vi "N4_X01_write_range.vi"(0 "DriverConnect in":T1={"InterfaceType"=enum."VISA", "OpenedSession"="", "InterfaceSettings"={"Interface"=enum."RS232", "EOS 4 read"=enum."LF (\\n)", "EOS 4 write"=enum."LF (\\n)", "TMO, ms"=10000, "Sett"=variant(cluster{"Baud Rate":u32, "Data Bits":u16, "Parity":u16, "Stop Bits":u16, "Flow Control":u16, "Eho":bool} {"Baud Rate"=75, "Data Bits"=0, "Parity"=0, "Stop Bits"=0, "Flow Control"=0, "Eho"=FALSE})}}, 1 "Command range":T7, 2 "ModeIsChanged?":T6, 11 "error in":T8, 12 "Error Code":T10, 14 "Driver Name":T9) -> (4 "DriverConnect out":T1={"InterfaceType"=enum."VISA", "OpenedSession"="", "InterfaceSettings"={"Interface"=enum."RS232", "EOS 4 read"=enum."LF (\\n)", "EOS 4 write"=enum."LF (\\n)", "TMO, ms"=10000, "Sett"=variant(cluster{"Baud Rate":u32, "Data Bits":u16, "Parity":u16, "Stop Bits":u16, "Flow Control":u16, "Eho":bool} {"Baud Rate"=75, "Data Bits"=0, "Parity"=0, "Stop Bits"=0, "Flow Control"=0, "Eho"=FALSE})}}, 8 "RangeWasChanged":T6=TRUE, 15 "error out":T8)   [LabVIEW 2018]
uses:
  MOKO_LabViewLibrary/MokoLowLevel/MokoLowLovelControl/MLLC_ErrorCode.ctl
  MOKO_LabViewLibrary/MokoLowLevel/MokoLowLovelControl/MLLC_DriverName.ctl
  MOKO_LabViewLibrary/MokoLowLevel/MokoLowLovelControl/MLLC_Error.ctl
  MOKO_LabViewLibrary/MokoLowLevel/MokoLowLovelControl/MLLC_Command.ctl
  MOKO_LabViewLibrary/MokoLowLevel/MokoLowLovelControl/MLLC_Boolean.ctl
  MOKO_LabViewLibrary/MokoLowLevel/MokoLowLovelControl/MLLC_ConnectCluster.ctl
  MOKO_LabViewLibrary/MokoLowLevel/MokoLowLovelControl/MLLC_InterfaceType.ctl
  MOKO_LabViewLibrary/MokoLowLevel/MokoLowLovelControl/MLLC_OpenedSession.ctl
  MOKO_LabViewLibrary/MokoLowLevel/MokoLowLovelControl/MLLC_InterfaceSettings.ctl
  MOKO_LabViewLibrary/MokoLowLevel/MokoLowLovelControl/MLLC_InterfaceKind.ctl
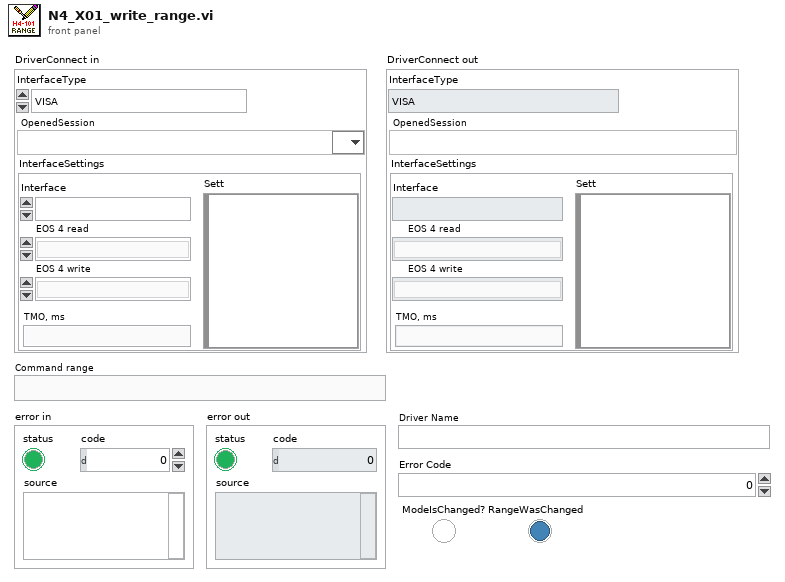
[diagram p1: front panel]
types:
  T1 = typedef "MLLC_ConnectCluster.ctl" = cluster{"InterfaceType":T2, "OpenedSession":T3, "InterfaceSettings":T4}
  T2 = typedef "MLLC_InterfaceType.ctl" = enum16{"VISA", "Prologix USB-GPIB"}
  T3 = typedef "MLLC_OpenedSession.ctl" = refnum<visa-resource-name>
  T4 = typedef "MLLC_InterfaceSettings.ctl" = cluster{"Interface":T5, "EOS 4 read":enum16{"Default (=EOS 4 write)", "CR (\\r)", "LF (\\n)", "None"}, "EOS 4 write":enum16{"CR+LF (\\r\\n)", "CR (\\r)", "LF (\\n)", "None"}, "TMO, ms":i32, "Sett":variant}
  T5 = typedef "MLLC_InterfaceKind.ctl" = enum16{"RS232", "GPIB", "USB", "Ethernet", "another"}
  T6 = typedef "MLLC_Boolean.ctl" = bool
  T7 = typedef "MLLC_Command.ctl" = string
  T8 = typedef "MLLC_Error.ctl" = errorcluster
  T9 = typedef "MLLC_DriverName.ctl" = string
  T10 = typedef "MLLC_ErrorCode.ctl" = u32
  T11 = typedef "MLLC_Response.ctl" = string
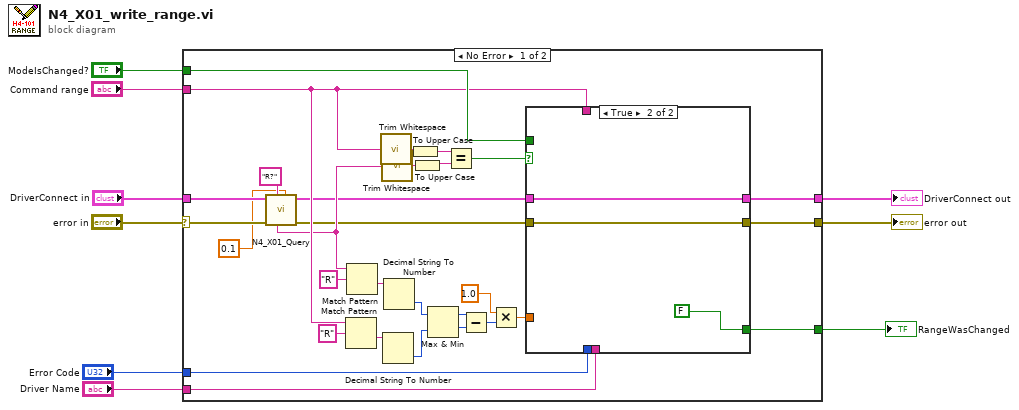
[diagram p0: block diagram]
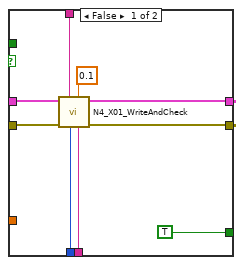
[diagram p2: hidden frame]
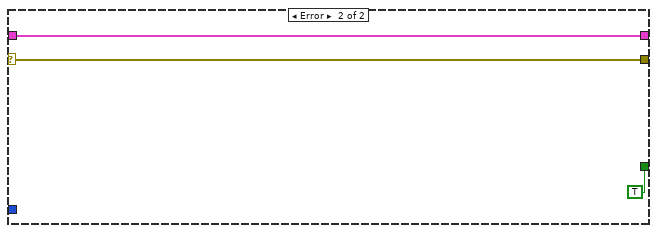
[diagram p3: hidden frame]
diagram:
  n1 = case shown="No Error" "error in" {
    selector: "error in" -> [w35 w54]
    tunnel: [w37 w54] -> w9
    tunnel: [w38 w53] -> w1
    tunnel: "Error Code" -> [w34 _]
    tunnel: "Driver Name" -> [w33 _]
    tunnel: "DriverConnect in" -> [w39 w53]
    tunnel: "Command range" -> [w31 _]
    tunnel: [w36 TRUE] -> w4
    tunnel: "ModeIsChanged?" -> [w32 _]
    frame No Error {
      n2 = call "N4_X01_Query.vi"("Delay Befor (s)"=0.1 ("Command Time (s)"), "Command"="R?" ("Error Query"), "error in"=w35, "DriverConnect in"=w39) -> ("error out"=w11:T8, "DriverConnect out"=w12:T1, "Response"=w13:T11)  [unwired: 5 in]
      n3 = Match Pattern(string=w31, regular expression="R") -> (after substring=w22:T7)  [unwired: 1 in, 3 out]
      n4 = Match Pattern(string=w13, regular expression="R") -> (after substring=w23:T11)  [unwired: 1 in, 3 out]
      n5 = call <vilib>:"Trim Whitespace.vi"("string"=w31) -> ("trimmed string"=w26:string)  [unwired: 1 in]
      n6 = call <vilib>:"Trim Whitespace.vi"("string"=w13) -> ("trimmed string"=w28:string)  [unwired: 1 in]
      n7 = Decimal String To Number(string=w22) -> (number=w19:i32)  [unwired: 2 in, 1 out]
      n8 = Decimal String To Number(string=w23) -> (number=w20:i32)  [unwired: 2 in, 1 out]
      n9 = To Upper Case(1:w26) -> (0:w27:string)
      n10 = To Upper Case(1:w28) -> (0:w29:string)
      n11 = Max & Min(x=w20, y=w19) -> (max(x,y)=w18:i32, min(x,y)=w17:i32)
      n12 = Equal?(x=w27, y=w29) -> (x = y?=w25:bool)
      n13 = Subtract(x=w18, y=w17) -> (x-y=w16:i32)
      n14 = Multiply(x=1.0 ("Delay Time (s)"), y=w16) -> (x*y=w15:dbl)
      n15 = case shown="True" w25 {
        tunnel: w34 -> [w48 _]
        tunnel: w33 -> [w47 _]
        tunnel: [w46 w51] -> w38
        tunnel: [w45 w50] -> w37
        tunnel: w31 -> [w44 _]
        tunnel: w12 -> [w41 w51]
        tunnel: w11 -> [w40 w50]
        tunnel: [TRUE FALSE] -> w36
        tunnel: w32 -> [_ _]
        tunnel: w15 -> [_ _]
        frame False {
          n16 = call "N4_X01_WriteAndCheck.vi"("Driver Name"=w47, "Command Time (s)"=0.1, "Error Code"=w48, "Command"=w44, "error in"=w40, "DriverConnect in"=w41) -> ("error out"=w45:T8, "DriverConnect out"=w46:T1)  [unwired: 4 in]
        }
        frame True {
        }
      }
    }
    frame Error {
    }
  }
  "error out" <- w9
  "RangeWasChanged" <- w4
  "DriverConnect out" <- w1
